vi "Create DAT File.vi"(8 "error in":errorcluster, 9 "DAT file name":string="8 - sweep B, Vsg IV.dat", 10 "Processed data folder":path=path "G:/My Drive/ansom/Data/MNK/SA03018F.20180124/processed", 11 "Retrieve and Visualize":refnum<class "Retrieve and Visualize.lvclass">) -> (0 "error out":errorcluster, 3 "Retrieve and Visualize out":refnum<class "Retrieve and Visualize.lvclass">)   [LabVIEW 2020, in "Retrieve and Visualize.lvclass"]
uses:
  Retrieve and Visualize.lvclass
  Retrieve and Visualize.lvclass/Retrieve and Visualize.ctl
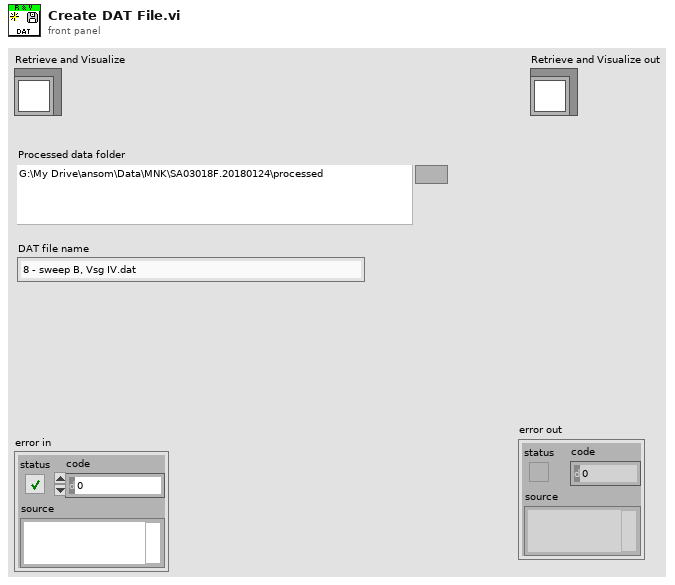
[diagram p1: front panel]
types:
  T1 = enum16{"open", "replace", "create", "open or create", "replace or create", "replace or create with confirmation"}
  T2 = cluster{"IV":cluster{dbl[], dbl[]}[][][], "IV-2T":cluster{dbl[], dbl[]}[][][], "Vfast":dbl[][], "Vslow":dbl[], "Vslowest":dbl[], "Comments":string, "Scan names":string[]}
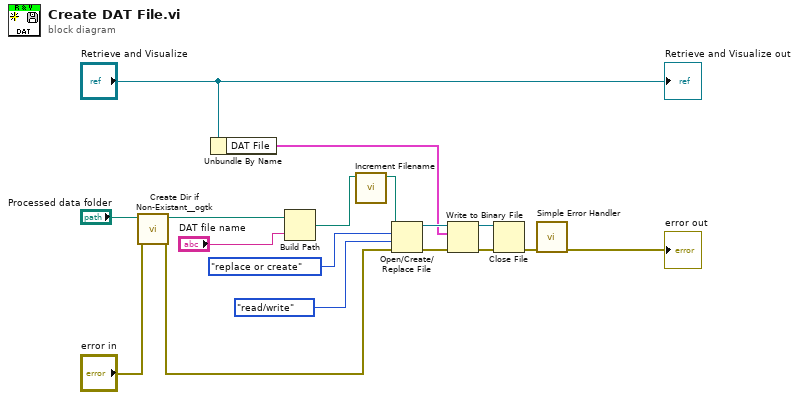
[diagram p0: block diagram]
diagram:
  n1 = call <userlib>:"Create Dir if Non-Existant__ogtk.vi"("error in (no error)"="error in", "Directory Path"="Processed data folder") -> ("error out"=w5:errorcluster, "dup Directory Path"=w4:path)  [unwired: 7 in, 1 out]
  n2 = Unbundle By Name("Retrieve and Visualize") -> ("DAT File"=w11:T2)
  n3 = Build Path(base path=w4, name or relative path="DAT file name") -> (appended path=w2:path)
  n4 = call <userlib>:"Increment Filename.vi"("Path"=w2) -> ("Modified Path"=w1:path)  [unwired: 9 in, 1 out]
  n5 = Open/Create/Replace File(file path (use dialog)=w1, error in=w5, operation (0:open)=T1."replace or create", access (0:read/write)=enum16{"read/write", "read-only", "write-only"}."read/write") -> (refnum out=w17:refnum<file>, error out=w16:errorcluster)  [unwired: 2 in, 1 out]
  n6 = Write to Binary File(file (use dialog)=w17, data=w11, error in=w16) -> (refnum out=w13:refnum<file>, error out=w14:errorcluster)  [unwired: 3 in, 1 out]
  n7 = Close File(refnum=w13, error in=w14) -> (error out=w15:errorcluster)  [unwired: 1 out]
  n8 = call <vilib>:"Simple Error Handler.vi"("error in (no error)"=w15) -> ("error out"=→"error out":errorcluster)  [unwired: 4 in, 4 out]
  "Retrieve and Visualize out" <- "Retrieve and Visualize"
